vi "Beta_Ver 1.0.vi"() -> ()   [LabVIEW 2015]
uses:
  <instrlib>/Keithley 622x LV 2009/Configure/Units/Typedefs/KE622x -- Voltage Meas Units.ctl
  <instrlib>/Keithley 622x LV 2009/Configure/2182 -A/Low Level/Typedefs/KE2182 -- Voltage Ranges.ctl
  <instrlib>/Keithley 622x LV 2009/Configure/2182 -A/Low Level/Typedefs/KE2182 -- Filter Type.ctl
  <instrlib>/Keithley 622x LV 2009/Configure/2182 -A/Low Level/Typedefs/KE2182 -- Filter Count.ctl
  <instrlib>/Keithley 622x LV 2009/Configure/2182 -A/Low Level/Typedefs/KE2182 -- Filter Window.ctl
  <instrlib>/Keithley 622x LV 2009/Configure/2182 -A/Low Level/Typedefs/KE2182 -- NPLCs.ctl
  <instrlib>/Keithley 622x LV 2009/Configure/Units/Typedefs/KE6221 -- PDelta Power Meas Type.ctl
  <instrlib>/Keithley 622x LV 2009/Configure/Delta PDelta DCon Modes/Typedefs/KE6221 -- PDelta Mode Params.ctl
  <instrlib>/Keithley 622x LV 2009/Configure/Delta PDelta DCon Modes/Low Level/Typedefs/KE622x -- Delta PDelta Mode High Level.ctl
  <instrlib>/Keithley 622x LV 2009/Configure/Delta PDelta DCon Modes/Low Level/Typedefs/KE622x -- Delta PDelta Mode Low Level.ctl
  <instrlib>/Keithley 622x LV 2009/Configure/Delta PDelta DCon Modes/Low Level/Typedefs/KE6221 -- PDelta Mode Pulse Width.ctl
  <instrlib>/Keithley 622x LV 2009/Configure/Delta PDelta DCon Modes/Low Level/Typedefs/KE6221 -- PDelta Mode Source Delay.ctl
  <instrlib>/Keithley 622x LV 2009/Configure/Delta PDelta DCon Modes/Low Level/Typedefs/KE622x -- Delta PDelta Mode Num Cycles Mode.ctl
  <instrlib>/Keithley 622x LV 2009/Configure/Delta PDelta DCon Modes/Low Level/Typedefs/KE622x -- Delta PDelta Mode Num Cycles.ctl
  <instrlib>/Keithley 622x LV 2009/Configure/Delta PDelta DCon Modes/Low Level/Typedefs/KE6221 -- PDelta Mode Ranging Mode.ctl
  <instrlib>/Keithley 622x LV 2009/Configure/Delta PDelta DCon Modes/Low Level/Typedefs/KE6221 -- PDelta Mode Num Low Meas.ctl
  <instrlib>/Keithley 622x LV 2009/Configure/Delta PDelta DCon Modes/Low Level/Typedefs/KE6221 -- PDelta Mode Pulse Period.ctl
  <instrlib>/Keithley 622x LV 2009/Configure/Format/Typedefs/KE622x -- Optional Meas Elements.ctl
  <instrlib>/Keithley 622x LV 2009/Configure/Trace Buf/Low Level/Typedefs/KE622x -- Trace Buf.ctl
  <instrlib>/Keithley 622x LV 2009/Configure/Delta PDelta DCon Modes/Low Level/Typedefs/KE622x -- Delta DCon Mode Delay.ctl
  <instrlib>/Keithley 622x LV 2009/Configure/Delta PDelta DCon Modes/Typedefs/KE622x -- Delta Mode Params.ctl
  <instrlib>/Keithley 622x LV 2009/Utility/Typedefs/KE622x -- Instrument Type.ctl
  <instrlib>/Keithley 622x LV 2009/Keithley 622x.lvlib
panel:
  out "COMMAND":string
  out "High Level (A)":T1=0.001 min=0.0 max=0.105 format="%.3e"
  out "Low Level (A)":T2=-0.001 min=-0.105 max=0.0 format="%.3e"
  out "Delay (s)":T3=0.002 min=0.001 max=9999.999 format="%.3f"
  out "Num Cycles Mode":T4
  out "Finite Count":T5=10 min=2 max=65536
  out "Abort On Compliance?":bool
  out "Cold Swithing Mode Enabled?":bool
  out "HI_L_COM":string
  out "LOW_L_COM":string
  out "COUN_COM":string
  out "COMP_COM":string
  out "COLD_COM":string
  out "DEL_COM":string
  out "FILE":refnum<file>
  out "Reading":sgl[](array[numeric])
  out "Trace Buf":T6 {"Average Voltage (V)" format="%.3p"; "Source Val (A)" format="%.3p"; "Timestamp (secs)" format="%.3f"; "Reading" format="%.7f"}
  in  "Meas Elements To Return":T7={"Timstamp?"=TRUE, "Reading Num?"=TRUE, "Source Value?"=FALSE, "Compliance?"=FALSE, "Average Voltage?"=FALSE}
  in  "stop":bool
  in  "Check For SCPI Errors? (T)":bool=TRUE
  in  "Power Meas Type":T8
  in  "2812 -A Params In":T14={"Auto Range?"=FALSE, "Man / Selected\nRange"=enum."10V", "Enable Digital\nFilter?"=FALSE, "Filter Type"=enum."Moving", "Filter Count"=10, "Filter\nWindow (%)"=0.01, "Enable Analog\nFilter?"=FALSE, "NPLCs"=5} {"Filter\nWindow (%)" min=0.0 max=10.0 step=0.01 format="%.2f"; "Filter Count" min=1 max=100; "NPLCs" min=1 max=10}
  in  "Measurement Units":T15
  in  "Measurements control":enum32{"PULSE", " DELTA"}(tab)
  in  "Pulsed Delta Mode Params In":T16={"High Level (A)"=0.001, "Low Level (A)"=0.0, "Pulse Width (s)"=0.00011, "Source Delay (s)"=1.6e-05, "Num Cycles Mode"=enum."Infinite", "Finite Count"=1, "Ranging Mode"=enum."Best", "Num Low Meas Per Cycle"=enum."2", "Pulse Period (Num PLCs)"=5, "Pulse Sweep Mode Enabled?"=FALSE} {"Pulse Period (Num PLCs)" min=5 max=999990; "Source Delay (s)" min=1.6e-05 max=0.011966 format="%.3p"; "Pulse Width (s)" min=5e-05 max=0.012 format="%.3p"; "Finite Count" min=2 max=65536; "Low Level (A)" min=-0.105 max=0.0 format="%.3p"; "High Level (A)" min=0.0 max=0.105 format="%.3p"}
  in  "Delta Mode Params In":T22={"High Level (A)"=0.001, "Low Level (A)"=-0.001, "Delay (s)"=0.002, "Num Cycles Mode"=enum."Finite Count", "Finite Count"=1, "Abort On\nCompliance?"=FALSE, "Cold Swithing\nMode Enabled?"=FALSE} {"Finite Count" min=1 max=65536; "Low Level (A)" min=-0.105 max=0.0 format="%.3p"; "High Level (A)" min=0.0 max=0.105 format="%.3p"; "Delay (s)" min=0.001 max=9999.999 format="%.3f"}
  in  "Comments":string
  in  "Folder \nPrename":string
  # "Keithley  6221 & 2182A Measurement System"
  # "FILE CONFIGURATION"
  # "PRE EXPERIMENT CONFIGS"
  # "*** NOTE:  \"Average Voltage\"\nis only available for Differential\nConductance measurements."
  # "*** NOTE:  \"Average Voltage\"\nis only available for Differential\nConductance measurements."
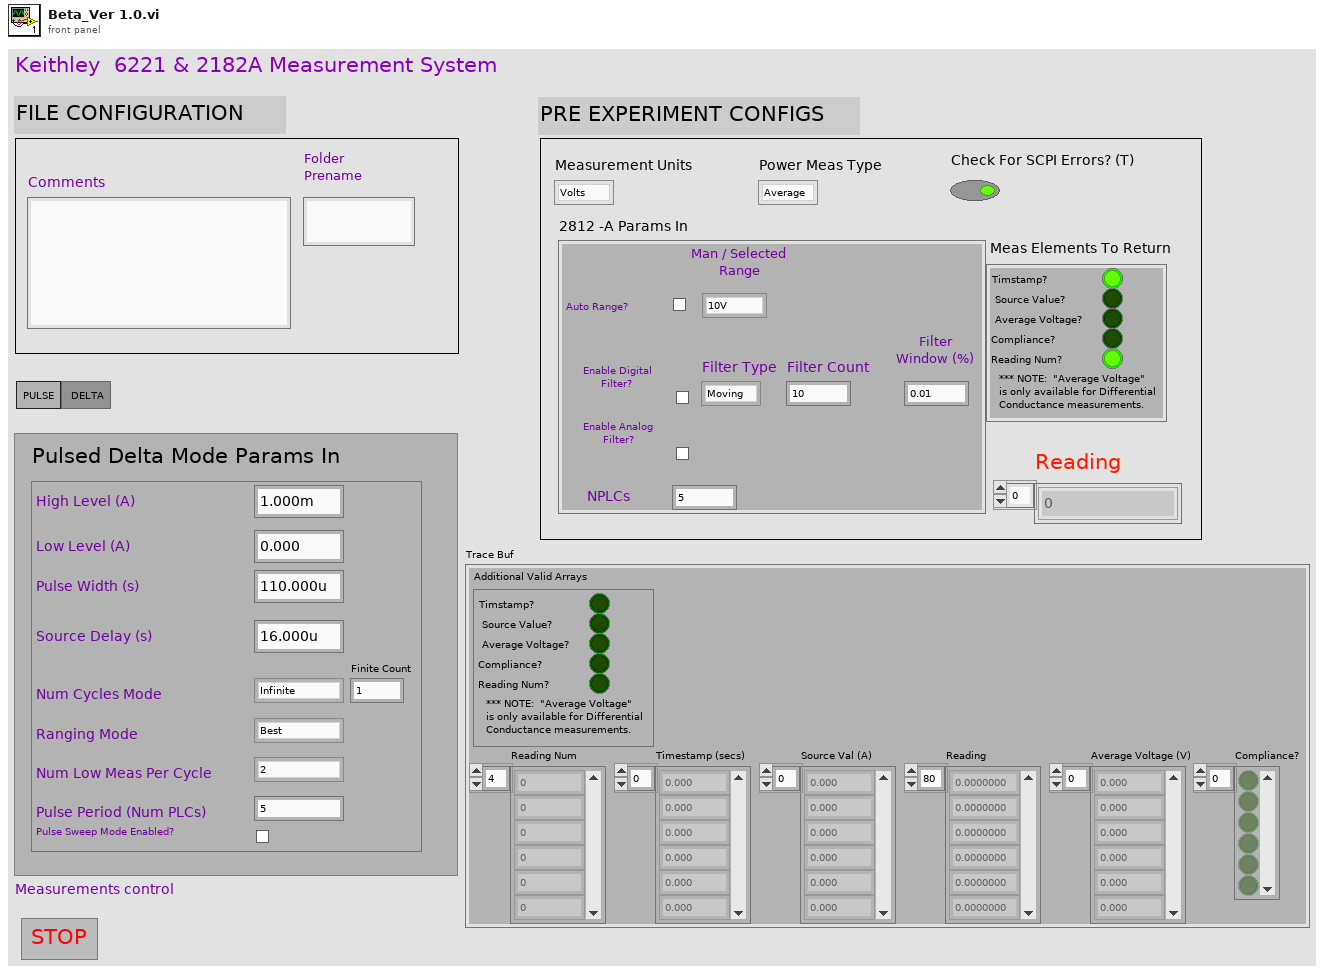
[diagram p1: front panel]
types:
  T1 = typedef "Keithley 622x.lvlib/KE622x -- Delta PDelta Mode High Level.ctl" = dbl
  T2 = typedef "Keithley 622x.lvlib/KE622x -- Delta PDelta Mode Low Level.ctl" = dbl
  T3 = typedef "Keithley 622x.lvlib/KE622x -- Delta DCon Mode Delay.ctl" = dbl
  T4 = typedef "Keithley 622x.lvlib/KE622x -- Delta PDelta Mode Num Cycles Mode.ctl" = enum16{"Finite Count", "Infinite"}
  T5 = typedef "Keithley 622x.lvlib/KE622x -- Delta PDelta Mode Num Cycles.ctl" = u32
  T6 = typedef "Keithley 622x.lvlib/KE622x -- Trace Buf.ctl" = cluster{"Additional Valid Arrays":T7, "Reading Num":u32[], "Timestamp (secs)":sgl[], "Source Val (A)":sgl[], "Reading":sgl[], "Average Voltage (V)":sgl[], "Compliance?":bool[]}
  T7 = typedef "Keithley 622x.lvlib/KE622x -- Optional Meas Elements.ctl" = cluster{"Timstamp?":bool, "Reading Num?":bool, "Source Value?":bool, "Compliance?":bool, "Average Voltage?":bool}
  T8 = typedef "Keithley 622x.lvlib/KE6221 -- PDelta Power Meas Type.ctl" = enum16{"Average", "Peak"}
  T9 = typedef "Keithley 622x.lvlib/KE2182 -- Voltage Ranges.ctl" = enum16{"10mV", "100mV", "1V", "10V", "100V"}
  T10 = typedef "Keithley 622x.lvlib/KE2182 -- Filter Type.ctl" = enum16{"Moving", "Repeat"}
  T11 = typedef "Keithley 622x.lvlib/KE2182 -- Filter Count.ctl" = u32
  T12 = typedef "Keithley 622x.lvlib/KE2182 -- Filter Window.ctl" = dbl
  T13 = typedef "Keithley 622x.lvlib/KE2182 -- NPLCs.ctl" = u32
  T14 = cluster{"Auto Range?":bool, "Man / Selected\nRange":T9, "Enable Digital\nFilter?":bool, "Filter Type":T10, "Filter Count":T11, "Filter\nWindow (%)":T12, "Enable Analog\nFilter?":bool, "NPLCs":T13}
  T15 = typedef "Keithley 622x.lvlib/KE622x -- Voltage Meas Units.ctl" = enum16{"Volts", "Ohms", "Watts", "Siemens"}
  T16 = typedef "Keithley 622x.lvlib/KE6221 -- PDelta Mode Params.ctl" = cluster{"High Level (A)":T1, "Low Level (A)":T2, "Pulse Width (s)":T17, "Source Delay (s)":T18, "Num Cycles Mode":T4, "Finite Count":T5, "Ranging Mode":T19, "Num Low Meas Per Cycle":T20, "Pulse Period (Num PLCs)":T21, "Pulse Sweep Mode Enabled?":bool}
  T17 = typedef "Keithley 622x.lvlib/KE6221 -- PDelta Mode Pulse Width.ctl" = dbl
  T18 = typedef "Keithley 622x.lvlib/KE6221 -- PDelta Mode Source Delay.ctl" = dbl
  T19 = typedef "Keithley 622x.lvlib/KE6221 -- PDelta Mode Ranging Mode.ctl" = enum16{"Best", "Fixed"}
  T20 = typedef "Keithley 622x.lvlib/KE6221 -- PDelta Mode Num Low Meas.ctl" = enum16{"1", "2"}
  T21 = typedef "Keithley 622x.lvlib/KE6221 -- PDelta Mode Pulse Period.ctl" = u32
  T22 = typedef "Keithley 622x.lvlib/KE622x -- Delta Mode Params.ctl" = cluster{"High Level (A)":T1, "Low Level (A)":T2, "Delay (s)":T3, "Num Cycles Mode":T4, "Finite Count":T5, "Abort On\nCompliance?":bool, "Cold Swithing\nMode Enabled?":bool}
  T23 = typedef "Keithley 622x.lvlib/KE622x -- Instrument Type.ctl" = enum16{"KE6220", "KE6221"}
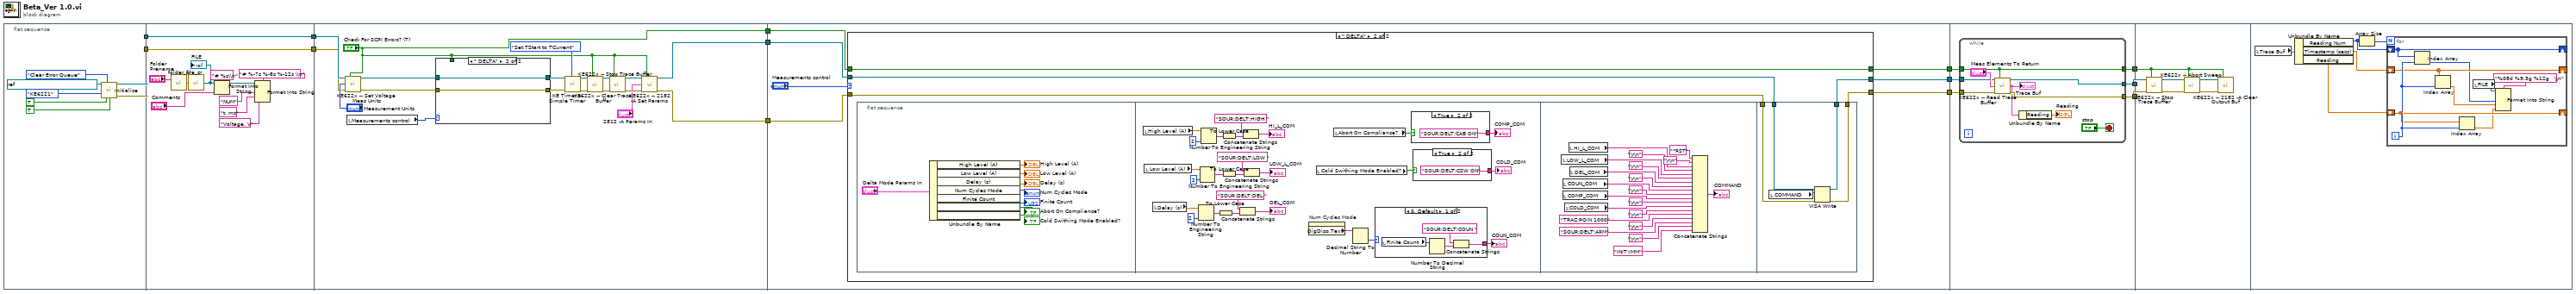
[diagram p0: block diagram]
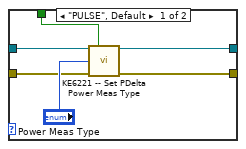
[diagram p2: hidden frame]
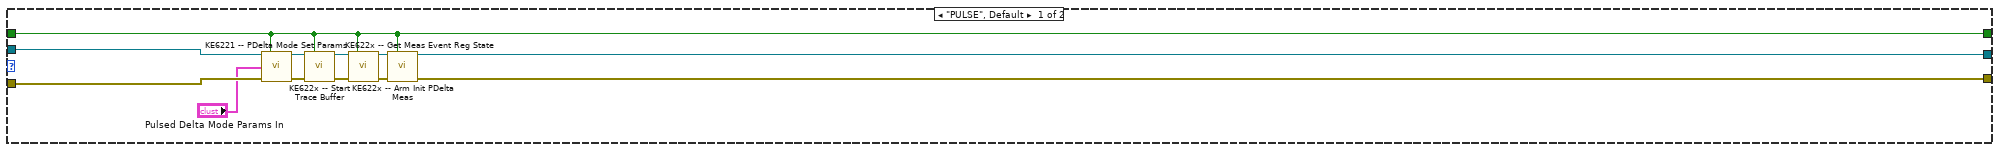
[diagram p3: hidden frame]
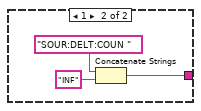
[diagram p4: hidden frame]
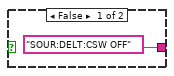
[diagram p5: hidden frame]
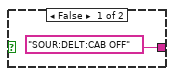
[diagram p6: hidden frame]
diagram:
  n1 = flat-sequence {
    tunnel: [w15] -> w4
    tunnel: [w14] -> w2
    tunnel: w4 -> [w32]
    tunnel: [w32] -> w3
    tunnel: w2 -> [w31]
    tunnel: [w31] -> w1
    tunnel: w3 -> [w50]
    tunnel: w1 -> [w49]
    tunnel: [w40] -> w13
    tunnel: [w39] -> w12
    tunnel: ["Check For SCPI Errors? (T)"] -> w11
    tunnel: w13 -> [w64]
    tunnel: w12 -> [w65]
    tunnel: w11 -> [w63]
    tunnel: [w62] -> w10
    tunnel: [w61] -> w9
    tunnel: [w60] -> w8
    tunnel: w10 -> [w158]
    tunnel: w9 -> [w157]
    tunnel: w8 -> [w156]
    tunnel: [w155] -> w7
    tunnel: [w154] -> w6
    tunnel: [w153] -> w5
    tunnel: w7 -> [w170]
    tunnel: w6 -> [w169]
    tunnel: w5 -> [w168]
    frame #0 {
      n2 = call <instrlib>:"Initialize.vi"("VISA resource name"=refnum<visa-resource-name> "DC_AC_Current_Source_6221", "Error Queue Option"=enum16{"Clear Error Queue", "Error Query"}."Clear Error Queue", "Instrument Type"=KE622x_--_Instrument_Type."KE6221", "ID Query? (T)"=TRUE, "Reset? (T)"=TRUE) -> ("VISA resource name out"=w15:refnum<visa-resource-name>, "error out"=w14:errorcluster)  [unwired: 9 in]
    }
    frame #1 {
      n3 = call "folder_cr.vi"("Name"="Folder \nPrename") -> ("String"=w23:string)
      n4 = call "file_cr.vi"("String"=w23) -> ("refnum out"=w21:refnum<file>)
      "FILE" <- w21
      n5 = Format Into String(format string="# %s\\n", initial string=w21, "Comments") -> (resulting string=w28:refnum<file>)  [unwired: 1 in, 1 out]
      n6 = Format Into String(format string="# %-7s %-8s %-12s \\n", initial string=w28, "NUM" ("input 1"), "t, ms" ("input 2"), "Voltage, V" ("input 3")) -> ()  [unwired: 1 in, 2 out]
    }
    frame #2 {
      n7 = call <instrlib>:"KE622x -- Set Voltage Meas Units.vi"("Resource In"=w50, "Check For SCPI Errors? (T)"="Check For SCPI Errors? (T)", "Voltage Meas Units"="Measurement Units", "error in (no error)"=w49) -> ("Resource Out (dupl)"=w36:refnum<visa-resource-name>, "error out"=w35:errorcluster)  [unwired: 10 in]
      n8 = local read "Measurements control"() -> (w38:enum32{"PULSE", " DELTA"})
      n9 = case shown="\" DELTA\"" w38 {
        tunnel: "Check For SCPI Errors? (T)" -> [w56 _]
        tunnel: w36 -> [w55 w59]
        tunnel: w35 -> [w54 w58]
        tunnel: [w53 w59] -> w34
        tunnel: [w52 w58] -> w33
        frame "PULSE", Default {
          n10 = call <instrlib>:"KE6221 -- Set PDelta Power Meas Type.vi"("6221 Resource In"=w55, "Check For SCPI Errors? (T)"=w56, "Power Meas Type"="Power Meas Type", "error in (no error)"=w54) -> ("6221 Resource Out (dupl)"=w53:refnum<visa-resource-name>, "error out"=w52:errorcluster)  [unwired: 10 in]
        }
        frame " DELTA" {
        }
      }
      n11 = call <instrlib>:"KE Timer -- Simple Timer.vi"("Resource In"=w34, "error in (no error)"=w33, "Action"=enum16{"Set TStart to TCurrent", "Get Deltas"}."Set TStart to TCurrent") -> ("Resource Out (dupl)"=w47:refnum<visa-resource-name>, "error out (dupl)"=w46:errorcluster)  [unwired: 7 in, 8 out]
      n12 = call <instrlib>:"KE622x -- Stop Trace Buffer.vi"("Resource In"=w47, "Check For SCPI Errors? (T)"="Check For SCPI Errors? (T)", "error in (no error)"=w46) -> ("Resource Out (dupl)"=w45:refnum<visa-resource-name>, "error out"=w44:errorcluster)  [unwired: 11 in]
      n13 = call <instrlib>:"KE622x -- Clear Trace Buffer.vi"("Resource In"=w45, "Check For SCPI Errors? (T)"="Check For SCPI Errors? (T)", "error in (no error)"=w44) -> ("Resource Out (dupl)"=w43:refnum<visa-resource-name>, "error out"=w42:errorcluster)  [unwired: 11 in]
      n14 = call <instrlib>:"KE622x -- 2182 -A Set Params.vi"("622x Resource In"=w43, "Check For SCPI Errors? (T)"="Check For SCPI Errors? (T)", "2812 -A Params In"="2812 -A Params In", "error in (no error)"=w42) -> ("622x Resource Out (dupl)"=w40:refnum<visa-resource-name>, "error out"=w39:errorcluster)  [unwired: 9 in, 1 out]
    }
    frame #3 {
      n15 = case shown="\" DELTA\"" "Measurements control" {
        tunnel: w65 -> [w77 w81]
        tunnel: w64 -> [w78 w82]
        tunnel: w63 -> [w67 w83]
        tunnel: [w69 w80] -> w62
        tunnel: [w68 w79] -> w61
        tunnel: [w67 w83] -> w60
        frame "PULSE", Default {
          n16 = call <instrlib>:"KE6221 -- PDelta Mode Set Params.vi"("6221 Resource In"=w78, "Check For SCPI Errors? (T)"=w67, "Pulsed Delta Mode Params In"="Pulsed Delta Mode Params In", "error in (no error)"=w77) -> ("6221 Resource Out (dupl)"=w75:refnum<visa-resource-name>, "error out"=w74:errorcluster)  [unwired: 9 in, 1 out]
          n17 = call <instrlib>:"KE622x -- Start Trace Buffer.vi"("Resource In"=w75, "Check For SCPI Errors? (T)"=w67, "error in (no error)"=w74) -> ("Resource Out (dupl)"=w73:refnum<visa-resource-name>, "error out"=w72:errorcluster)  [unwired: 11 in]
          n18 = call <instrlib>:"KE622x -- Get Meas Event Reg State.vi"("VISA Resource In"=w73, "Error Query (T)?"=w67, "error in (no error)"=w72) -> ("VISA Resource Out (dupl)"=w71:refnum<visa-resource-name>, "error out"=w70:errorcluster)  [unwired: 10 in, 1 out]
          n19 = call <instrlib>:"KE622x -- Arm Init PDelta Meas.vi"("Resource In"=w71, "Check For SCPI Errors? (T)"=w67, "error in (no error)"=w70) -> ("Resource Out (dupl)"=w69:refnum<visa-resource-name>, "error out"=w68:errorcluster)  [unwired: 11 in]
        }
        frame " DELTA" {
          n20 = flat-sequence {
            tunnel: w82 -> [w152]
            tunnel: w81 -> [w151]
            tunnel: [w149] -> w80
            tunnel: [w148] -> w79
            frame #0 {
              n21 = Unbundle By Name("Delta Mode Params In") -> ("High Level (A)"=→"High Level (A)":T1, "Low Level (A)"=→"Low Level (A)":T2, "Delay (s)"=→"Delay (s)":T3, "Num Cycles Mode"=→"Num Cycles Mode":T4, "Finite Count"=→"Finite Count":T5, "Abort On\nCompliance?"=→"Abort On Compliance?":bool, "Cold Swithing\nMode Enabled?"=→"Cold Swithing Mode Enabled?":bool)
            }
            frame #1 {
              n22 = local read "High Level (A)"() -> (w115:T1)
              n23 = local read "Low Level (A)"() -> (w114:T2)
              n24 = local read "Delay (s)"() -> (w111:T3)
              n25 = Number To Engineering String(2:i16 2 ("precision (6)"), 4:w111) -> (0:w100:string)  [unwired: 2 in]
              n26 = Number To Engineering String(2:i16 2 ("precision (6)"), 4:w114) -> (0:w102:string)  [unwired: 2 in]
              n27 = Number To Engineering String(2:i16 2 ("precision (6)"), 4:w115) -> (0:w103:string)  [unwired: 2 in]
              n28 = To Lower Case(string=w100) -> (all lower case string=w99:string)
              n29 = To Lower Case(string=w103) -> (all lower case string=w104:string)
              n30 = To Lower Case(string=w102) -> (all lower case string=w101:string)
              n31 = Concatenate Strings("SOUR:DELT:DEL " ("string"), w99) -> (→"DEL_COM":string)
              n32 = Concatenate Strings("SOUR:DELT:HIGH " ("string"), w104) -> (→"HI_L_COM":string)
              n33 = Concatenate Strings("SOUR:DELT:LOW " ("string"), w101) -> (→"LOW_L_COM":string)
              n34 = property on="Num Cycles Mode" class="Enum (strict)"() -> ("DigDisp.Text"=w94:string)  [unwired: 2 in, 2 out]
              n35 = local read "Cold Swithing Mode Enabled?"() -> (w95:bool)
              n36 = local read "Abort On Compliance?"() -> (w96:bool)
              n37 = Decimal String To Number(string=w94) -> (number=w93:i32)  [unwired: 2 in, 1 out]
              n38 = case shown="0, Default" w93 {
                tunnel: [w117 w121] -> w92
                frame 0, Default {
                  n39 = local read "Finite Count"() -> (w119:T5)
                  n40 = Number To Decimal String(number=w119) -> (decimal integer string=w118:string)  [unwired: 1 in]
                  n41 = Concatenate Strings("SOUR:DELT:COUN " ("string"), w118) -> (w117:string)
                }
                frame 1 {
                  n42 = Concatenate Strings("SOUR:DELT:COUN " ("string"), "INF" ("string")) -> (w121:string)
                }
              }
              "COUN_COM" <- w92
              n43 = case shown="True" w96 {
                tunnel: ["SOUR:DELT:CAB OFF" ("string") "SOUR:DELT:CAB ON" ("string")] -> w98
                frame False {
                }
                frame True {
                }
              }
              "COMP_COM" <- w98
              n44 = case shown="True" w95 {
                tunnel: ["SOUR:DELT:CSW OFF" ("string") "SOUR:DELT:CSW ON" ("string")] -> w97
                frame False {
                }
                frame True {
                }
              }
              "COLD_COM" <- w97
            }
            frame #2 {
              n45 = local read "LOW_L_COM"() -> (w140:string)
              n46 = local read "COUN_COM"() -> (w142:string)
              n47 = local read "COMP_COM"() -> (w143:string)
              n48 = local read "COLD_COM"() -> (w144:string)
              n49 = local read "HI_L_COM"() -> (w139:string)
              n50 = local read "DEL_COM"() -> (w141:string)
              n51 = Concatenate Strings("*RST" ("string"), "\r\n", w139, "\r\n", w140, "\r\n", w141, "\r\n", w142, "\r\n", w143, "\r\n", w144, "\r\n", "TRAC:POIN 1000" ("string"), "\r\n", "SOUR:DELT:ARM" ("string"), "\r\n", "INIT:IMM" ("string")) -> (→"COMMAND":string)
            }
            frame #3 {
              n52 = local read "COMMAND"() -> (w150:string)
              n53 = VISA Write(VISA resource name=w152, write buffer=w150, error in (no error)=w151) -> (VISA resource name out=w149:refnum<visa-resource-name>, error out=w148:errorcluster)  [unwired: 1 out]
            }
          }
        }
      }
    }
    frame #4 {
      n54 = while {
        tunnel: w158 -> [w164]
        tunnel: w157 -> [w165]
        tunnel: w156 -> [w163]
        tunnel: [w163] -> w155
        tunnel: [w162] -> w154
        tunnel: [w161] -> w153
        stop <- "stop" stop-if-true
        n55 = call <instrlib>:"KE622x -- Read Trace Buffer.vi"("Resource In"=w164, "Check For SCPI Errors? (T)"=w163, "Meas Elements To Return"="Meas Elements To Return", "error in (no error)"=w165) -> ("Resource Out (dupl)"=w162:refnum<visa-resource-name>, "Trace Buf"=w160:T6, "error out"=w161:errorcluster)  [unwired: 9 in]
        "Trace Buf" <- w160
        n56 = Unbundle By Name(w160) -> ("Reading"=→"Reading":sgl[])
      }
    }
    frame #5 {
      n57 = call <instrlib>:"KE622x -- Stop Trace Buffer.vi"("Resource In"=w169, "Check For SCPI Errors? (T)"=w170, "error in (no error)"=w168) -> ("Resource Out (dupl)"=w174:refnum<visa-resource-name>, "error out"=w172:errorcluster)  [unwired: 11 in]
      n58 = call <instrlib>:"KE622x -- Abort Sweep.vi"("Resource In"=w174, "Check For SCPI Errors? (T)"=w170, "error in (no error)"=w172) -> ("Resource Out (dupl)"=w173:refnum<visa-resource-name>, "error out"=w171:errorcluster)  [unwired: 11 in]
      n59 = call <instrlib>:"KE622x -- 2182 -A Clear Output Buf.vi"("622x Resource In"=w173, "Check For SCPI Errors? (T)"=w170, "error in (no error)"=w171) -> ()  [unwired: 10 in, 3 out]
    }
    frame #6 {
      n60 = local read "Trace Buf"() -> (w179:T6)
      n61 = Unbundle By Name(w179) -> ("Reading Num"=w175:u32[], "Timestamp (secs)"=w177:sgl[], "Reading"=w176:sgl[])
      n62 = Array Size(array=w175) -> (size(s)=w178:i32)
      n63 = for {
        N: w178 -> [_]
        shift-right: [w187] -> _
        shift-left: w175 -> [w187]
        shift-right: [w186] -> _
        shift-left: w177 -> [w186]
        shift-right: [w185] -> _
        shift-left: w176 -> [w185]
        i -> [w188]
        n64 = Index Array(array=w187, index=w188) -> (element=w182:u32)
        n65 = Index Array(array=w186, index=w188) -> (element=w181:sgl)
        n66 = Index Array(array=w185, index=w188) -> (element=w180:sgl)
        n67 = local read "FILE"() -> (w184:refnum<file>)
        n68 = Format Into String(format string="%08d %9.3g %12g   \\n", initial string=w184, w182, w181, w180) -> ()  [unwired: 1 in, 2 out]
      }
    }
  }
